vi "Calibration Cal Execute RF Test Get Default Parameters.vi"(8 "error in (no error)":errorcluster, 11 "Template Tx Test in":refnum<class "niDTS Calibration Cal Execute RF Test.lvclass">) -> (0 "error out":errorcluster, 2 "Parameters":T1={"Calibration Mode"=2} {"Calibration Mode" items=["Full", "If Needed"]}, 3 "Template Tx Test out":refnum<class "niDTS Calibration Cal Execute RF Test.lvclass">)   [LabVIEW 2015, in "niDTS Utilities.lvlib" / "niDTS Calibration Cal Execute RF Test.lvclass"]
uses:
  niDTS Calibration Cal Execute RF Test.lvclass
  Includes/niDTS Calibration Cal Execute RF Test INC Parameters.ctl
  niDTS Utilities.lvlib
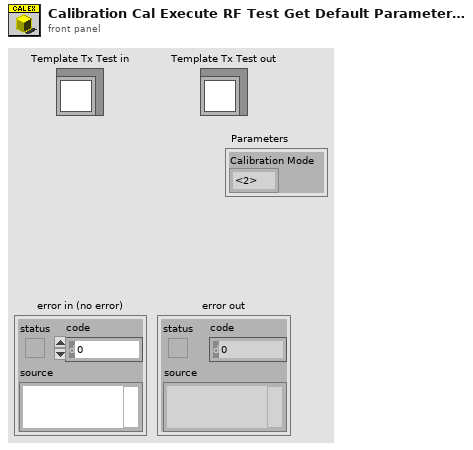
[diagram p1: front panel]
types:
  T1 = typedef "niDTS Utilities.lvlib/niDTS Calibration Cal Execute RF Test INC Parameters.ctl" = cluster{"Calibration Mode":u16}
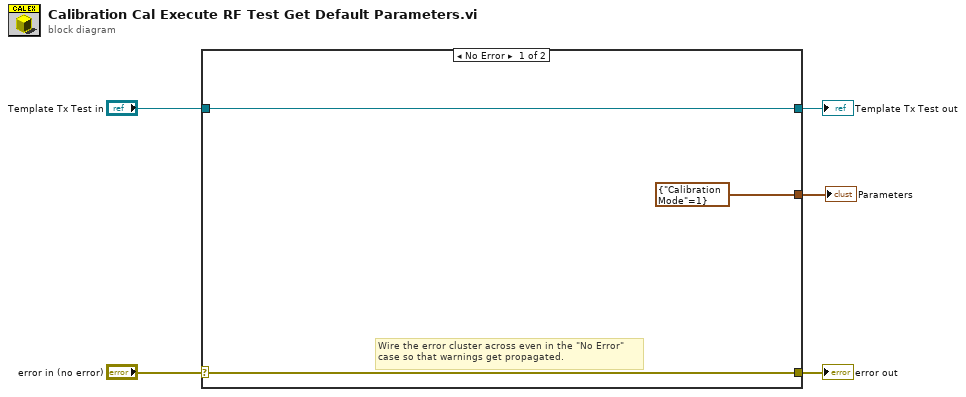
[diagram p0: block diagram]
diagram:
  n1 = case shown="No Error" "error in (no error)" {
    selector: "error in (no error)" -> [w8 w10]
    tunnel: [w8 w10] -> w4
    tunnel: [w7 w9] -> w2
    tunnel: "Template Tx Test in" -> [w7 w9]
    tunnel: [T1 {"Calibration Mode"=1} ("Parameters") _] -> w1
    frame No Error {
      # "Wire the error cluster across even in the \"No Error\"\ncase so that warnings get propagated."
    }
    frame Error {
    }
  }
  "error out" <- w4
  "Template Tx Test out" <- w2
  "Parameters" <- w1
